vi "Connection Events.vi"() -> ()   [LabVIEW 2018]
uses:
  TwinCAT ADS Class/Controls/Connection Information.ctl
  TwinCAT ADS Class/Controls/Address.ctl
  TwinCAT ADS Class/Controls/Connection Protocol.ctl
  TwinCAT ADS Class/Controls/Router State.ctl
  TwinCAT ADS Class/Controls/Connection State.ctl
  TwinCAT ADS Class/TwinCAT ADS.lvclass/TwinCAT ADS.ctl
  TwinCAT ADS Class/TwinCAT ADS.lvclass
panel:
  in  "Disconnect":bool
  in  "Connect":bool
  out "Connection Information":T1
  in  "stop":bool
  # "Change AMS Router\nby reactivating TwinCAT System \nwhist this VI is running to get \nAMS events"
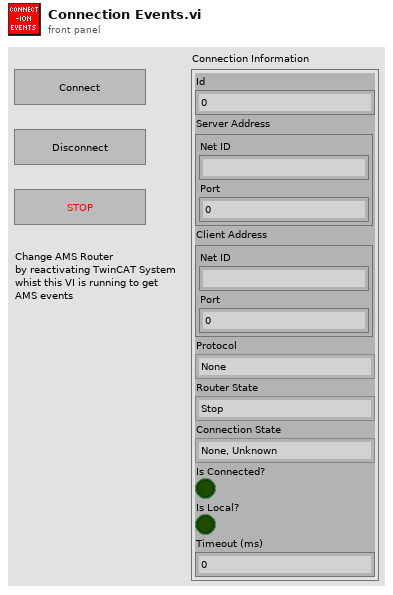
[diagram p1: front panel]
types:
  T1 = typedef "TwinCAT ADS.lvclass/Connection Information.ctl" = cluster{"Id":i32, "Server Address":T2, "Client Address":cluster{"Net ID":string, "Port":i32}, "Protocol":T3, "Router State":T4, "Connection State":T5, "Is Connected?":bool, "Is Local?":bool, "Timeout (ms)":i32}
  T2 = typedef "TwinCAT ADS.lvclass/Address.ctl" = cluster{"Net ID":string, "Port":i32}
  T3 = typedef "TwinCAT ADS.lvclass/Connection Protocol.ctl" = enum16{"None", "Router", "TCP/IP", "All"}
  T4 = typedef "TwinCAT ADS.lvclass/Router State.ctl" = enum16{"Stop", "Start", "Removed", "Unknown"}
  T5 = typedef "TwinCAT ADS.lvclass/Connection State.ctl" = enum16{"None, Unknown", "Disconnected", "Connected", "Lost"}
  T6 = enum16{"None, Unknown", "Disconnected", "Connected", "Lost"}
  T7 = enum16{"None", "Established", "Closed", "Lost", "Error", "Resurrected"}
  T8 = enum16{"Invalid", "Idle", "Reset", "Init", "Start", "Run", "Stop", "SaveConfig", "LoadConfig", "PowerFailure", "PowerGood", "Error", "Shutdown", "Suspend", "Resume", "Config", "Reconfig", "Stopping, Maxstates", "Incompatible", "Exception"}
  T9 = typedef "TwinCAT ADS.lvclass/AMS Router State.ctl" = enum32{"Stop", "Start", "Removed", "Unknown"}
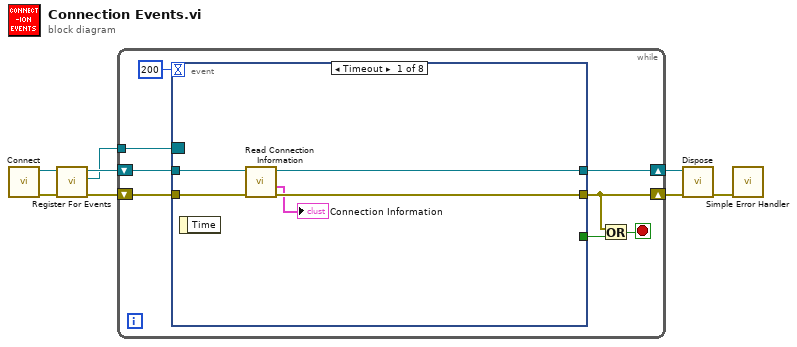
[diagram p0: block diagram]
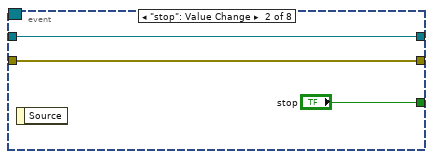
[diagram p2: hidden frame]
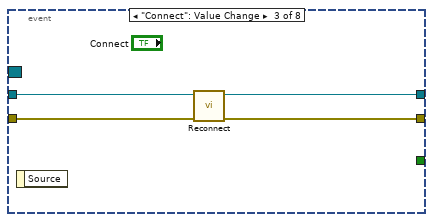
[diagram p3: hidden frame]
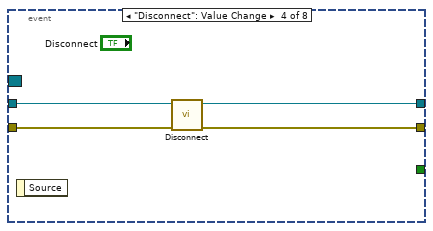
[diagram p4: hidden frame]
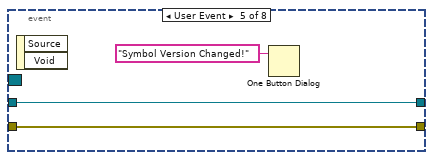
[diagram p5: hidden frame]
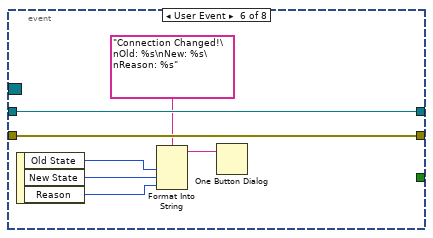
[diagram p6: hidden frame]
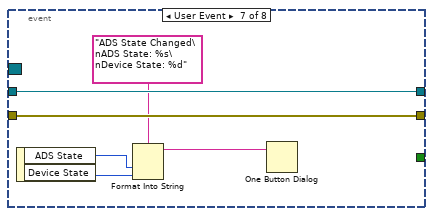
[diagram p7: hidden frame]
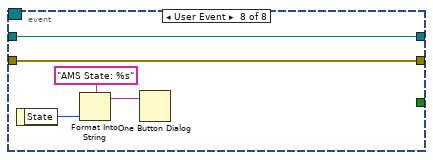
[diagram p8: hidden frame]
diagram:
  n1 = call "Connect.vi"() -> ("error out"=w1:errorcluster, "TwinCAT ADS out"=w2:refnum<class "TwinCAT ADS.lvclass">)  [unwired: 10 in]
  n2 = call "Register For Events.vi"("error in (no error)"=w1, "TwinCAT ADS in"=w2) -> ("error out"=w5:errorcluster, "Event Registration Refnum"=w3:refnum<event-registration>, "TwinCAT ADS out"=w4:refnum<class "TwinCAT ADS.lvclass">)  [unwired: 7 in]
  n3 = while {
    shift-right: [w14] -> w7
    shift-left: w4 -> [w16]
    shift-right: [w11] -> w6
    shift-left: w5 -> [w15]
    tunnel: w3 -> [w9]
    stop <- w12 stop-if-true
    n4 = event shown="[0] Timeout" {
      selector: w9 -> [_ _ _ _ _ _ _ _]
      dyn-events: _ -> [_ _ _ _ _ _ _ _]
      timeout: 200 -> [_ _ _ _ _ _ _ _]
      tunnel: w16 -> [w21 w24 w28 w32 w35 w42 w48 w53]
      tunnel: w15 -> [w20 w23 w27 w31 w34 w41 w47 w52]
      tunnel: [w18 w24 w26 w29 w35 w42 w48 w53] -> w14
      tunnel: [w19 w23 w25 w30 w34 w41 w47 w52] -> w11
      tunnel: [_ "stop" _ _ _ _ _ _] -> w10
      event Timeout {
        n5 = event-data() -> ()  [unwired: 1 in, 1 out]
        n6 = call "Read Connection Information.vi"("error in (no error)"=w20, "TwinCAT ADS in"=w21) -> ("error out"=w19:errorcluster, "Connection Information"=→"Connection Information":T1, "TwinCAT ADS out"=w18:refnum<class "TwinCAT ADS.lvclass">)  [unwired: 7 in]
      }
      event "stop": Value Change {
        n7 = event-data() -> ()  [unwired: 1 in, 1 out]
      }
      event "Connect": Value Change {
        n8 = event-data() -> ()  [unwired: 1 in, 1 out]
        n9 = call "Reconnect.vi"("error in (no error)"=w27, "TwinCAT ADS in"=w28) -> ("error out"=w25:errorcluster, "TwinCAT ADS out"=w26:refnum<class "TwinCAT ADS.lvclass">)  [unwired: 8 in]
      }
      event "Disconnect": Value Change {
        n10 = event-data() -> ()  [unwired: 1 in, 1 out]
        n11 = call "Disconnect.vi"("error in (no error)"=w31, "TwinCAT ADS in"=w32) -> ("error out"=w30:errorcluster, "TwinCAT ADS out"=w29:refnum<class "TwinCAT ADS.lvclass">)  [unwired: 7 in, 1 out]
      }
      event User Event {
        n12 = event-data() -> ()  [unwired: 1 in, 2 out]
        n13 = One Button Dialog(message="Symbol Version Changed!") -> ()  [unwired: 1 in, 1 out]
      }
      event User Event {
        n14 = event-data() -> ("Old State"=w40:T6, "New State"=w39:T6, "Reason"=w38:T7)  [unwired: 1 in]
        n15 = Format Into String(format string="Connection Changed!\nOld: %s\nNew: %s\nReason: %s" ("message"), w40, w39, w38) -> (resulting string=w36:string)  [unwired: 2 in, 1 out]
        n16 = One Button Dialog(message=w36) -> ()  [unwired: 1 in, 1 out]
      }
      event User Event {
        n17 = event-data() -> ("ADS State"=w45:T8, "Device State"=w44:i16)  [unwired: 1 in]
        n18 = Format Into String(format string="ADS State Changed\nADS State: %s\nDevice State: %d" ("message"), w45, w44) -> (resulting string=w46:string)  [unwired: 2 in, 1 out]
        n19 = One Button Dialog(message=w46) -> ()  [unwired: 1 in, 1 out]
      }
      event User Event {
        n20 = event-data() -> ("State"=w50:T9)  [unwired: 1 in]
        n21 = Format Into String(format string="AMS State: %s" ("message"), w50) -> (resulting string=w51:string)  [unwired: 2 in, 1 out]
        n22 = One Button Dialog(message=w51) -> ()  [unwired: 1 in, 1 out]
      }
    }
    n23 = Or(x=w11, y=w10) -> (x .or. y?=w12:bool)
  }
  n24 = call "Dispose.vi"("error in (no error)"=w6, "TwinCAT ADS in"=w7) -> ("error out"=w8:errorcluster)  [unwired: 9 in]
  n25 = call <vilib>:"Simple Error Handler.vi"("error in (no error)"=w8) -> ()  [unwired: 4 in, 5 out]
